vi "SMU_Output Connected Config.vi"(7 "Output Connected":bool=TRUE, 8 "error in (no error)":errorcluster, 10 "Channel Lists":string[](array[string]), 11 "DCPower Sessions In":refnum<k15>[](array[refnum])) -> (0 "error Out":errorcluster, 3 "Instrument Sessions Out":refnum<k15>[](array[refnum]))   [LabVIEW 2013]
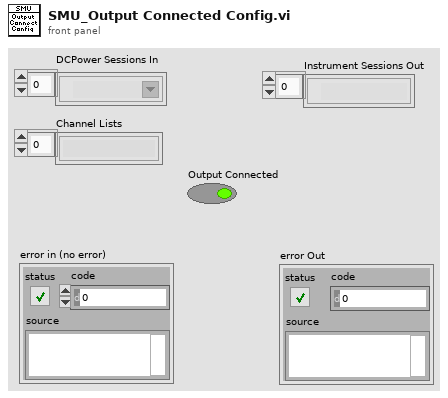
[diagram p1: front panel]
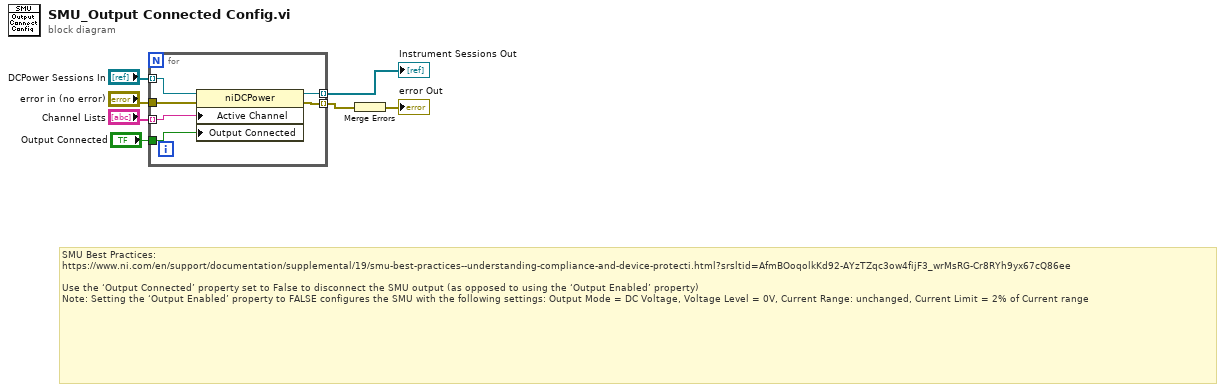
[diagram p0: block diagram]
diagram:
  # "SMU Best Practices:\nhttps://www.ni.com/en/support/documentation/supplemental/19/smu-best-practices--understanding-compliance-and-device-protecti.html?srsltid=AfmBOoqolkKd92-AYzTZqc3ow4fijF3_wrMsRG-Cr8RYh9yx67cQ86ee\n\nUse the ‘Output Connected’ property set to False to disconnect the SMU output (as opposed to using the ‘Output Enabled’ property)\nNote: Setting the ‘Output Enabled’ property to FALSE configures the SMU with the following settings: Output Mode = DC Voltage, Voltage Level = 0V, Current Range: unchanged, Current Limit = 2% of Current range"
  n1 = for {
    tunnel: "DCPower Sessions In" -> [w13] mode=indexing
    tunnel: "error in (no error)" -> [w12]
    tunnel: "Channel Lists" -> [w11] mode=indexing
    tunnel: "Output Connected" -> [w10]
    tunnel: [w9] -> w1 mode=indexing
    tunnel: [w8] -> w3 mode=indexing
    n2 = property class="niDCPower"(reference=w13, error in=w12, "Active Channel"=w11, "Output Connected"=w10) -> (reference out=w9:refnum<k15>, error out=w8:errorcluster)
  }
  "Instrument Sessions Out" <- w1
  n3 = Merge Errors(w3) -> (→"error Out":errorcluster)
